vi "DataFile_Append.vi"(8 "iteration":i32, 11 "DataCluster":T1={"Core"={"Current VI Reference"=refnum, "Close Panel on Exit?"=FALSE, "Exit"=FALSE, "Initialized?"=FALSE}, "Connections"={"cDAQ Therm"={"Task"="", "Connected"=FALSE, "Active"=FALSE}, "cDAQ Voltage"={"Task"="", "Connected"=FALSE, "Active"=FALSE}, "cDAQ ID"="", "Camera"={"Session"="", "Connected"=FALSE, "Active"=FALSE, "Placeholder"=refnum}, "PSU"={"Port"="", "Connected"=FALSE, "Active"=FALSE}}, "Data Acquisition"={"Setup"={"Label"="", "Operator"="", "Notes"="", "TempGrad"=1.0, "TargetTemp"=1.0, "Sample Volume"=1.0}, "Camera"={"Image"=refnum, "Save Image"=refnum, "Image Frequency"=20, "Rectangle"={"Left"=0, "Top"=0, "Right"=0, "Bottom"=0, "Rotation"=0.0}, "Calibration"={"Top Left"={"X"=0.0, "Y"=0.0}, "Top Right"={"X"=0.0, "Y"=0.0}, "Bottom Left"={"X"=0.0, "Y"=0.0}, "Bottom Right"={"X"=0.0, "Y"=0.0}, "Fixpoint"={"X"=0.0, "Y"=0.0}, "Scan Area"=0.0, "Fixpoint Area"=0.0, "Well Pixels"=[], "Valid"=FALSE}, "FocusPos"=0, "Display Mapping"=10}, "Thermistor"={"Sample Size"=1, "Calibration"={"B0.100"=[], "R25"=[], "c"=[], "State"=[], "V_S"=5.0, "R_S"=100.0}, "Timing Mode"=14713}, "Partition"={"Data"=[], "Cell Label"="", "Cell Color"=0, "Height"=10, "Width"=16, "Grid"=[]}, "Queue"={"Size"=1, "Queue"=refnum}, "Sample Rate"=1, "Active"=FALSE, "Ready"=FALSE, "Graph Mode"=0}, "Control"={"Sample Rate"=1, "PID gains"={"proportional gain (Kc)"=1.0, "integral time (Ti, min)"=0.01, "derivative time (Td, min)"=0.0}}} {"Control"."PID gains"."derivative time (Td, min)" format="%.3f"; "Control"."PID gains"."integral time (Ti, min)" format="%.3f"; "Control"."PID gains"."proportional gain (Kc)" format="%.3f"; "Control"."Sample Rate" min=1 max=20 step=1 format="%.0f Samples/sec"; "Data Acquisition"."Graph Mode" items=["Thermistor Temperature", "Camera Temperature"]; "Data Acquisition"."Thermistor"."Timing Mode" items=["Automatic"=16097, "High Resolution"=10195, "High Speed"=14712, "Best 50 Hz Rejection"=14713, "Best 60 Hz Rejection"=14714, "Custom"=10137]; "Data Acquisition"."Thermistor"."Calibration"."R_S" min=0.1 max=1000.0 format="%#_g kOhm"; "Data Acquisition"."Thermistor"."Calibration"."V_S" min=5.0 max=48.0 format="%#_g V"; "Data Acquisition"."Thermistor"."Calibration"."R25" min=0.1 max=1000.0 format="%#_g kOhm"; "Data Acquisition"."Thermistor"."Calibration"."B0.100" min=100.0 max=10000.0 format="%#_g K"; "Data Acquisition"."Thermistor"."Sample Size" min=1 max=200; "Data Acquisition"."Sample Rate" min=20 max=240 format="%.0f samples/min"; "Data Acquisition"."Queue"."Size" min=1 max=200; "Data Acquisition"."Camera"."Display Mapping" items=["Default"=10, "Most Significant Bits"=11, "Full Dynamic"=12, "Downshift"=13, "Given Range"=14, "90% Dynamic"=15, "Given Percent Range"=16]; "Data Acquisition"."Camera"."Calibration"."Fixpoint"."Y" format="%.2f"; "Data Acquisition"."Camera"."Calibration"."Fixpoint"."X" format="%.2f"; "Data Acquisition"."Camera"."Calibration"."Top Left"."Y" format="%.2f"; "Data Acquisition"."Camera"."Calibration"."Top Left"."X" format="%.2f"; "Data Acquisition"."Camera"."Calibration"."Top Right"."Y" format="%.2f"; "Data Acquisition"."Camera"."Calibration"."Top Right"."X" format="%.2f"; "Data Acquisition"."Camera"."Calibration"."Bottom Left"."Y" format="%.2f"; "Data Acquisition"."Camera"."Calibration"."Bottom Left"."X" format="%.2f"; "Data Acquisition"."Camera"."Calibration"."Bottom Right"."Y" format="%.2f"; "Data Acquisition"."Camera"."Calibration"."Bottom Right"."X" format="%.2f"; "Data Acquisition"."Camera"."Rectangle"."Rotation" min=-90.0 max=90.0 step=1.0 format="%.2f"; "Data Acquisition"."Camera"."Rectangle"."Left" scale=0.0..1024.0; "Data Acquisition"."Camera"."Rectangle"."Right" scale=0.0..1024.0; "Data Acquisition"."Camera"."Image Frequency" min=1 max=60 step=1; "Data Acquisition"."Setup"."Sample Volume" min=0.0 max=500.0 format="%#_g µL"; "Data Acquisition"."Setup"."TargetTemp" min=-40.0 max=40.0 step=0.5 format="%#_g °C"; "Data Acquisition"."Setup"."TempGrad" min=-100.0 max=100.0 step=0.1 format="%#_g °C/min"}) -> (0 "iteration out":i32)   [LabVIEW 2020]
uses:
  DataCluster.ctl
  <vilib>/userDefined/High Color/IMAQdx.ctl
  <vilib>/vision/Image Controls.llb/IMAQ Image.ctl
  <vilib>/Utility/file.llb/Write Delimited Spreadsheet (string).vi
panel:
  out "error out 2":errorcluster
  out "error out":errorcluster
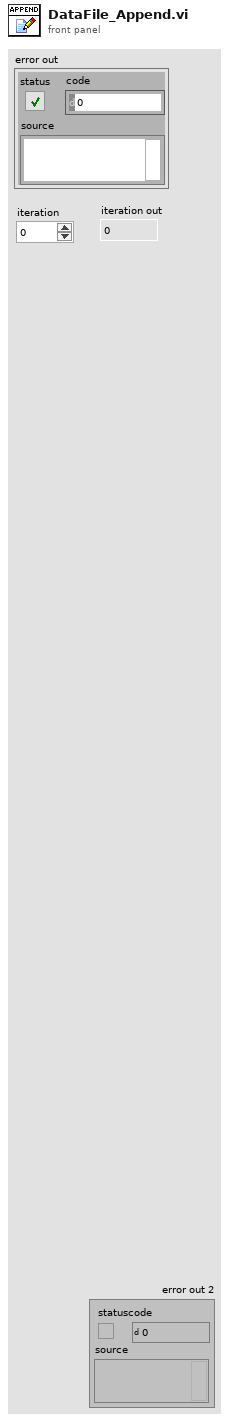
[diagram p1: front panel]
types:
  T1 = typedef "DataCluster.ctl" = cluster{"Core":cluster{"Current VI Reference":refnum<vi>, "Close Panel on Exit?":bool, "Exit":bool, "Initialized?":bool}, "Connections":cluster{"cDAQ Therm":cluster{"Task":refnum<k21>, "Connected":bool, "Active":bool}, "cDAQ Voltage":cluster{"Task":refnum<k21>, "Connected":bool, "Active":bool}, "cDAQ ID":string, "Camera":cluster{"Session":T2, "Connected":bool, "Active":bool, "Placeholder":T3}, "PSU":cluster{"Port":refnum<visa-resource-name>, "Connected":bool, "Active":bool}}, "Data Acquisition":cluster{"Setup":cluster{"Label":string, "Operator":string, "Notes":string, "TempGrad":dbl, "TargetTemp":dbl, "Sample Volume":dbl}, "Camera":cluster{"Image":T3, "Save Image":T3, "Image Frequency":i32, "Rectangle":T4, "Calibration":cluster{"Top Left":T5, "Top Right":T5, "Bottom Left":T5, "Bottom Right":T5, "Fixpoint":T5, "Scan Area":dbl, "Fixpoint Area":dbl, "Well Pixels":cluster{"X":i32, "Y":i32}[][], "Valid":bool}, "FocusPos":u32, "Display Mapping":u32}, "Thermistor":cluster{"Sample Size":i32, "Calibration":cluster{"B0.100":dbl[], "R25":dbl[], "c":dbl[][], "State":bool[], "V_S":dbl, "R_S":dbl}, "Timing Mode":i32}, "Partition":cluster{"Data":string[][], "Cell Label":string, "Cell Color":u32, "Height":i32, "Width":i32, "Grid":string[][]}, "Queue":cluster{"Size":i32, "Queue":refnum<queue>}, "Sample Rate":i32, "Active":bool, "Ready":bool, "Graph Mode":u16}, "Control":cluster{"Sample Rate":i32, "PID gains":cluster{"proportional gain (Kc)":dbl, "integral time (Ti, min)":dbl, "derivative time (Td, min)":dbl}}}
  T2 = typedef "IMAQdx.ctl" = refnum<k21>
  T3 = typedef "IMAQ Image.ctl" = refnum<image>
  T4 = typedef "IMAQ Rectangle" = cluster{"Left":i32, "Top":i32, "Right":i32, "Bottom":i32, "Rotation":dbl}
  T5 = typedef "IMAQ Point" = cluster{"X":sgl, "Y":sgl}
  T6 = cluster{"Mean Temperature":dbl, "Temp Gradient":dbl, "Temperature Readings":dbl[], "Voltage Readings":dbl[], "Temp Std":dbl[], "Image Pixels (U32)":u16[][], string}
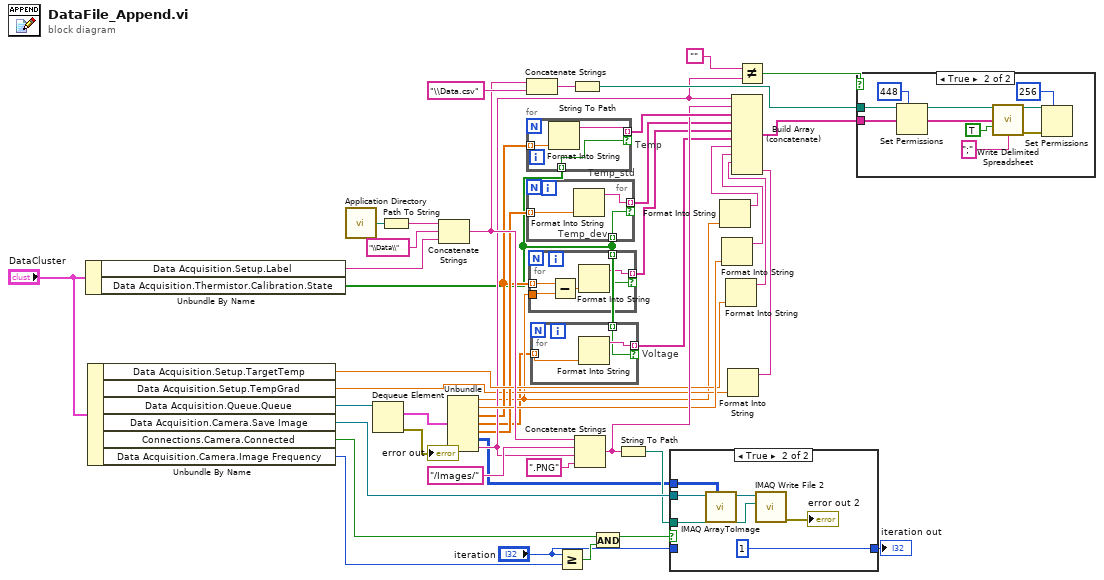
[diagram p0: block diagram]
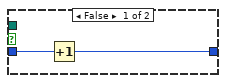
[diagram p3: hidden frame]
diagram:
  n1 = Unbundle By Name("DataCluster") -> ("Data Acquisition.Setup.Label"=w41:string, "Data Acquisition.Thermistor.Calibration.State"=w1:bool[])
  n2 = Unbundle By Name("DataCluster") -> ("Data Acquisition.Setup.TargetTemp"=w12:dbl, "Data Acquisition.Setup.TempGrad"=w7:dbl, "Data Acquisition.Queue.Queue"=w38:refnum<queue>, "Data Acquisition.Camera.Save Image"=w34:T3, "Connections.Camera.Connected"=w27:bool, "Data Acquisition.Camera.Image Frequency"=w20:i32)
  n3 = call <vilib>:"Application Directory.vi"() -> ("Application Directory"=w44:path)
  n4 = Dequeue Element(queue=w38) -> (element=w36:T6, error out=→"error out":errorcluster)  [unwired: 2 in, 2 out]
  n5 = Path To String(path=w44) -> (string=w43:string)
  n6 = Concatenate Strings(w43, "\\Data\\", w41) -> (w23:string)
  n7 = Unbundle(w36) -> ("Mean Temperature"=w6:dbl, "Temp Gradient"=w17:dbl, "Temperature Readings"=w8:dbl[], "Voltage Readings"=w5:dbl[], "Temp Std"=w9:dbl[], "Image Pixels (U32)"=w10:u16[][], w11:string)
  n8 = Concatenate Strings(w23, "\\Data.csv") -> (w33:string)
  n9 = for "Temp" {
    tunnel: w8 -> [w47] mode=indexing
    tunnel: [w46] -> w37 mode=indexing if=w45
    tunnel: w1 -> [w45] mode=indexing
    n10 = Format Into String(w47) -> (resulting string=w46:string)  [unwired: 3 in, 1 out]
  }
  n11 = for "Temp_std" {
    tunnel: w9 -> [w50] mode=indexing
    tunnel: [w49] -> w4 mode=indexing if=w48
    tunnel: w1 -> [w48] mode=indexing
    n12 = Format Into String(w50) -> (resulting string=w49:string)  [unwired: 3 in, 1 out]
  }
  n13 = for "Temp_dev" {
    tunnel: w8 -> [w55] mode=indexing
    tunnel: [w54] -> w3 mode=indexing if=w53
    tunnel: w1 -> [w53] mode=indexing
    tunnel: w6 -> [w51]
    n14 = Subtract(x=w55, y=w51) -> (x-y=w52:dbl)
    n15 = Format Into String(w52) -> (resulting string=w54:string)  [unwired: 3 in, 1 out]
  }
  n16 = for "Voltage" {
    tunnel: [w58] -> w2 mode=indexing if=w57
    tunnel: w1 -> [w57] mode=indexing
    tunnel: w5 -> [w56] mode=indexing
    n17 = Format Into String(w56) -> (resulting string=w58:string)  [unwired: 3 in, 1 out]
  }
  n18 = Greater Or Equal?(x="iteration", y=w20) -> (x >= y?=w21:bool)
  n19 = String To Path(string=w33) -> (path=w40:path)
  n20 = Concatenate Strings(w23, "/Images/" ("string"), w11, ".PNG" ("string")) -> (w28:string)
  n21 = And(x=w27, y=w21) -> (x .and. y?=w22:bool)
  n22 = String To Path(string=w28) -> (path=w30:path)
  n23 = case shown="True" w22 {
    tunnel: w10 -> [_ w61]
    tunnel: w34 -> [_ w63]
    tunnel: w30 -> [_ w66]
    tunnel: "iteration" -> [w60 _]
    tunnel: [w59 1] -> w18
    frame False {
      n24 = Increment(x=w60) -> (x+1=w59:i32)
    }
    frame True {
      n25 = call "IMAQ ArrayToImage"("Image Pixels (U16)"=w61, "Image"=w63) -> ("Image Out"=w62:T3)  [unwired: 8 in, 1 out]
      n26 = call-poly "IMAQ Write File 2"("File Path"=w66, "Image"=w62) -> ("error out"=→"error out 2":errorcluster)  [unwired: 8 in, 1 out]
    }
  }
  "iteration out" <- w18
  n27 = Format Into String(w6) -> (resulting string=w16:string)  [unwired: 3 in, 1 out]
  n28 = Format Into String(w17) -> (resulting string=w15:string)  [unwired: 3 in, 1 out]
  n29 = Format Into String(w12) -> (resulting string=w14:string)  [unwired: 3 in, 1 out]
  n30 = Format Into String(w7) -> (resulting string=w13:string)  [unwired: 3 in, 1 out]
  n31 = Build Array (concatenate)(w11, w28, w37, w4, w3, w2, w16, w15, w14, w13) -> (w29:string[])
  n32 = Not Equal?(x="", y=w11) -> (x != y?=w24:bool)
  n33 = case shown="True" w24 {
    tunnel: w40 -> [_ w72]
    tunnel: w29 -> [_ w73]
    frame False {
    }
    frame True {
      n34 = Set Permissions(7:i16 448 ("permissions"), 11:w72) -> (3:w71:path)  [unwired: 3 in, 1 out]
      n35 = call-poly <vilib>:"Write Delimited Spreadsheet.vi"("file path (dialog if empty)"=w71, "1D data"=w73, "append to file? (new file:F)"=TRUE, "delimiter (\\t)"=";" ("delimiter (\\t)")) -> ("new file path (Not A Path if cancelled)"=w70:path, "error out"=w69:errorcluster)  [unwired: 10 in]
      n36 = Set Permissions(7:i16 256 ("permissions"), 8:w69, 11:w70) -> ()  [unwired: 2 in, 2 out]
    }
  }
